vi "Exit.vi"(8 "error in (no error)":errorcluster) -> (0 "error out":errorcluster)   [LabVIEW 2018, in "Exit.lvlib"]
uses:
  Exit.lvlib
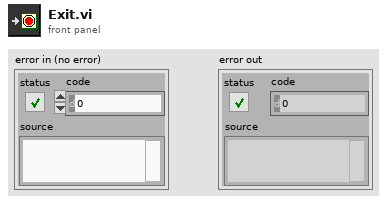
[diagram p1: front panel]
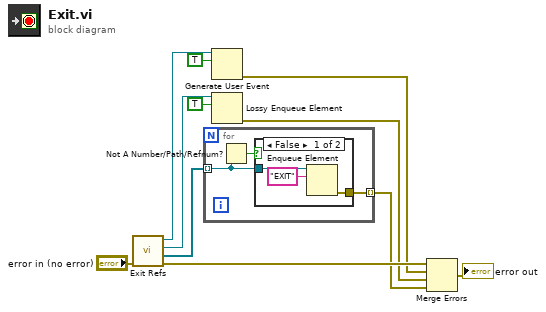
[diagram p0: block diagram]
diagram:
  n1 = call "Exit Refs.vi"("error in (no error)"="error in (no error)") -> ("error out"=w11:errorcluster, "Registered Queues"=w8:refnum<queue>[], "Exit SEQ"=w3:refnum<queue>, "Exit User Event"=w10:refnum<user-event>)  [unwired: 7 in]
  n2 = for {
    tunnel: w8 -> [w14] mode=indexing
    tunnel: [w12] -> w6 mode=indexing
    n3 = Not A Number/Path/Refnum?(number/path/refnum=w14) -> (NaN/Path/Refnum?=w13:bool)
    n4 = case shown="False" w13 {
      tunnel: w14 -> [w17 _]
      tunnel: [w15 _] -> w12
      frame False {
        n5 = Enqueue Element(queue=w17, element="EXIT") -> (error out=w15:errorcluster)  [unwired: 2 in, 2 out]
      }
      frame True {
      }
    }
  }
  n6 = Generate User Event(user event=w10, event data cluster=TRUE ("event data")) -> (error out=w7:errorcluster)  [unwired: 2 in, 1 out]
  n7 = Lossy Enqueue Element(queue=w3, element=TRUE) -> (error out=w1:errorcluster)  [unwired: 1 in, 3 out]
  n8 = Merge Errors(w11, w7, w1, w6) -> (→"error out":errorcluster)
